vi "no-so-random-data-array-generator.vi"(11 "Numeric in":dbl) -> (0 "data4":dbl format="%.2f", 2 "Array Out":dbl[](array[numeric]), 3 "Numeric out":dbl, 4 "data3":dbl format="%.2f", 6 "data2":dbl format="%.2f", 8 "data1":dbl format="%.2f")   [LabVIEW 2020]
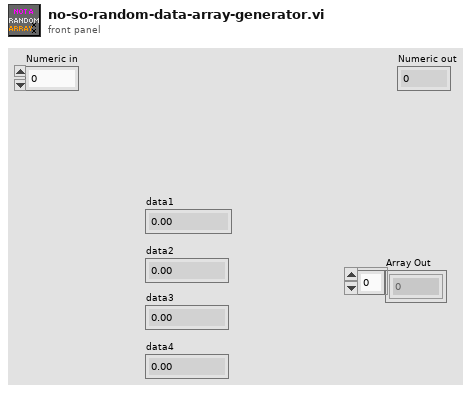
[diagram p1: front panel]
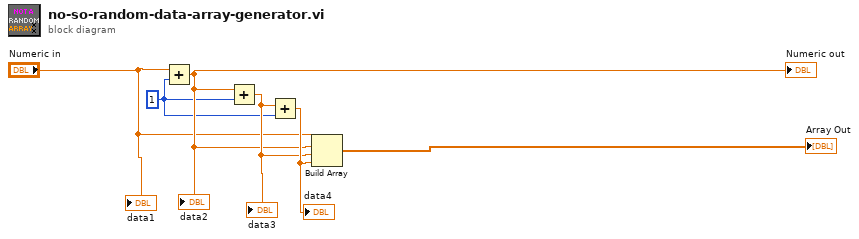
[diagram p0: block diagram]
diagram:
  w1 = 1 ("y")
  n1 = Add(x="Numeric in", y=w1) -> (x+y=w3:dbl)
  "data2" <- w3
  "Numeric out" <- w3
  n2 = Add(x=w3, y=w1) -> (x+y=w4:dbl)
  "data3" <- w4
  n3 = Add(x=w4, y=w1) -> (x+y=w5:dbl)
  "data4" <- w5
  n4 = Build Array("Numeric in", w3, w4, w5) -> (→"Array Out":dbl[])
  "data1" <- "Numeric in"
